vi "ProgramControlledDemo.vi"() -> ()   [LabVIEW 2016]
doc: "This VI shows how to setup and execute a measurement without any user input."
panel:
  out "LicenseIsValid":bool
  in  "Signal index to display":i32
  out "Diagram":waveform(dbl)(graph)
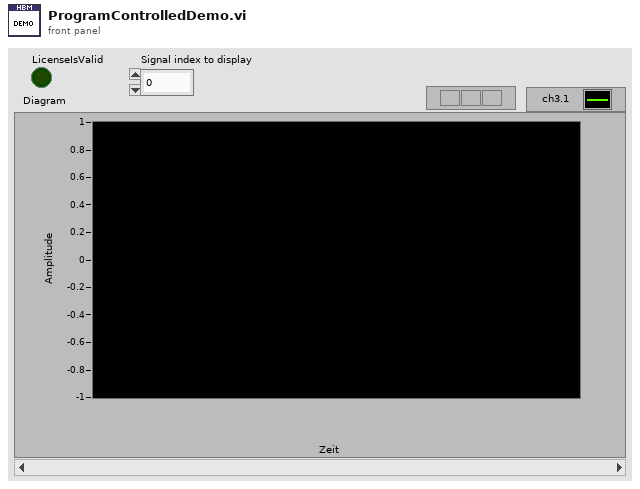
[diagram p1: front panel]
types:
  T1 = cluster{"Devices":refnum<k24>[], "Signals":refnum<k24>[]}
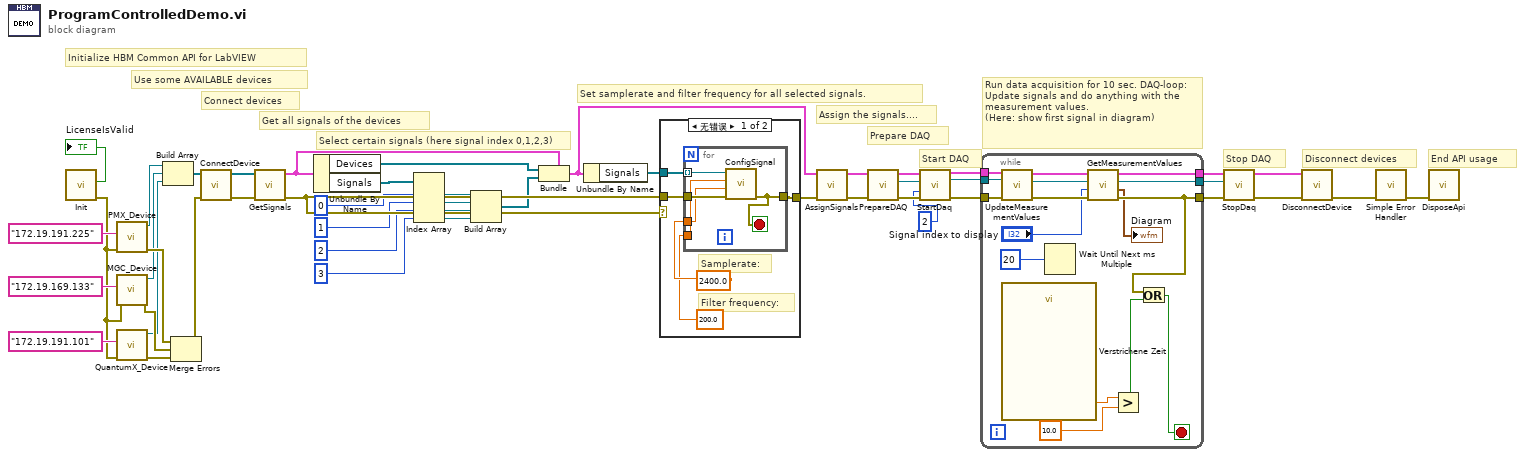
[diagram p0: block diagram]
diagram:
  # "Disconnect devices"
  # "Set samplerate and filter frequency for all selected signals."
  # "Initialize HBM Common API for LabVIEW"
  # "End API usage"
  # "Stop DAQ"
  # "Run data acquisition for 10 sec. DAQ-loop: Update signals and do anything with the  measurement values.\n(Here: show first signal in diagram)"
  # "Start DAQ"
  # "Prepare DAQ"
  # "Select certain signals (here signal index 0,1,2,3)"
  # "Get all signals of the devices"
  # "Connect devices"
  # "Use some AVAILABLE devices"
  # "Assign the signals...."
  n1 = call "Init.vi"() -> ("LicenseIsValid"=→"LicenseIsValid":bool, "Error out"=w27:errorcluster)  [unwired: 8 in, 1 out]
  n2 = call "PMX_Device.vi"("Error in"=w27, "IPAddress"="172.19.191.225") -> ("Error out"=w24:errorcluster, "Device"=w22:refnum<k24>)  [unwired: 8 in]
  n3 = call "MGC_Device.vi"("Error in"=w27, "IPAddress"="172.19.169.133") -> ("Error out"=w25:errorcluster, "Device"=w20:refnum<k24>)  [unwired: 8 in]
  n4 = call "QuantumX_Device.vi"("Error in"=w27, "IPAddress"="172.19.191.101") -> ("Error out"=w26:errorcluster, "Device"=w19:refnum<k24>)  [unwired: 6 in]
  n5 = Build Array(w22, w20, w19) -> (w21:refnum<k24>[])
  n6 = Merge Errors(w24, w25, w26) -> (w23:errorcluster)
  n7 = call "ConnectDevice.vi"("Error in"=w23, "Devices"=w21) -> ("Error out"=w34:errorcluster, "Devices"=w33:refnum<k24>[])  [unwired: 7 in, 1 out]
  n8 = call "GetSignals.vi"("Error in"=w34, "Devices"=w33) -> ("Error out"=w16:errorcluster, "DevicesAndSignals"=w17:T1)  [unwired: 7 in, 1 out]
  n9 = Unbundle By Name(w17) -> ("Devices"=w10:refnum<k24>[], "Signals"=w14:refnum<k24>[])
  n10 = Index Array(array=w14, index #1=0 ("Index"), index #2=1 ("Index"), index #3=2 ("Index"), index #4=3 ("Index")) -> (element #1=w13:refnum<k24>, element #2=w12:refnum<k24>, element #3=w5:refnum<k24>, element #4=w4:refnum<k24>)
  n11 = Build Array(w13, w12, w5, w4) -> (w11:refnum<k24>[])
  n12 = Bundle(cluster=w17, "Devices"=w10, "Signals"=w11) -> (w18:T1)
  n13 = Unbundle By Name(w18) -> ("Signals"=w47:refnum<k24>[])
  n14 = case shown="无错误" w16 {
    tunnel: w16 -> [w52 w58]
    tunnel: w47 -> [w51 _]
    tunnel: [w50 w58] -> w46
    frame No Error {
      # "Filter frequency:"
      # "Samplerate:"
      n15 = for {
        tunnel: w52 -> [w57]
        tunnel: 2400.0 ("SampleRate") -> [w56]
        tunnel: 200.0 ("FilterFrequency") -> [w55]
        tunnel: w51 -> [w54] mode=indexing
        tunnel: [w53] -> w50
        stop <- w53 stop-if-true
        n16 = call "ConfigSignal.vi"("Error in"=w57, "SampleRate"=w56, "FilterFrequency"=w55, "Signal"=w54) -> ("Error out"=w53:errorcluster)  [unwired: 7 in]
      }
    }
    frame Error {
    }
  }
  n17 = call "AssignSignals.vi"("Error in"=w46, "DevicesAndSignals"=w18) -> ("Error out"=w44:errorcluster, "DevicesAndSignals"=w45:T1)  [unwired: 8 in]
  n18 = call "PrepareDAQ.vi"("Error in"=w44, "DevicesAndSignals"=w45) -> ("Error out"=w41:errorcluster, "DaqMeasurement"=w42:refnum<k24>, "DevicesAndSignals"=w43:T1)  [unwired: 7 in]
  n19 = call "StartDaq.vi"("DevicesAndSignals"=w43, "DaqMeasurement"=w42, "AcquisitionMode"=2, "Error in"=w41) -> ("DevicesAndSignals"=w38:T1, "DaqMeasurement"=w39:refnum<k24>, "Error out"=w40:errorcluster)  [unwired: 8 in, 1 out]
  n20 = while {
    tunnel: w39 -> [w73]
    tunnel: w38 -> [w72]
    tunnel: [w67] -> w36
    tunnel: [w66] -> w35
    tunnel: w40 -> [w74]
    tunnel: [w63] -> w37
    stop <- w64 stop-if-true
    n21 = call "UpdateMeasurementValues.vi"("Error in"=w74, "DaqMeasurement"=w73, "DevicesAndSignals"=w72) -> ("Error out"=w69:errorcluster, "DaqMeasurement"=w70:refnum<k24>, "DevicesAndSignals"=w71:T1)  [unwired: 6 in]
    n22 = call "Verstrichene Zeit"() -> ("Elapsed Time (s)"=w61:dbl)  [unwired: 12 in, 7 out]
    n23 = Wait Until Next ms Multiple(millisecond multiple=u32 20 ("Vielfache von ms")) -> ()  [unwired: 1 out]
    n24 = call "GetMeasurementValues.vi"("Error in"=w69, "Index"="Signal index to display", "DaqMeasurement"=w70, "DevicesAndSignals"=w71) -> ("Error out"=w63:errorcluster, "Waveform"=→"Diagram":waveform(dbl), "DaqMeasurement"=w67:refnum<k24>, "DevicesAndSignals"=w66:T1)  [unwired: 4 in]
    n25 = Greater?(x=w61, y=10.0) -> (0:w59:bool)
    n26 = Or(x=w63, y=w59) -> (x .or. y?=w64:bool)
  }
  n27 = call "StopDaq.vi"("Error in"=w37, "DaqMeasurement"=w36, "DevicesAndSignals"=w35) -> ("Error out"=w3:errorcluster, "DevicesAndSignals"=w2:T1)  [unwired: 7 in]
  n28 = call "DisconnectDevice.vi"("Error in"=w3, "DevicesAndSignals"=w2) -> ("Error out"=w1:errorcluster)  [unwired: 9 in]
  n29 = call <vilib>:"Simple Error Handler.vi"("error in (no error)"=w1) -> ("error out"=w32:errorcluster)  [unwired: 4 in, 4 out]
  n30 = call "DisposeApi.vi"("Error in"=w32) -> ()  [unwired: 10 in, 1 out]
